vi "Page_Advanced_WriteAll.vi"(6 "ctl references":T1, 8 "error in (no error)":errorcluster, 11 "AB_InteropAssembly in":refnum<class "AB_InteropAssembly.lvclass">) -> (0 "error out":errorcluster, 3 "AB_InteropAssembly out":refnum<class "AB_InteropAssembly.lvclass">)   [LabVIEW 2020, in "AB_InteropAssembly.lvclass"]
uses:
  <vilib>/AppBuilder/AB_Classes/InteropAssembly/AB_InteropAssembly.lvclass
  <resource>/Framework/Providers/Builds/AppBuilder/AB_UI_Page_Advanced_References.ctl
  <vilib>/AppBuilder/AB_Classes/InteropAssembly/AB_InteropAssembly.lvclass/AB_InteropAssembly.ctl
  <vilib>/AppBuilder/AB_Classes/Application/AB_Application.lvclass
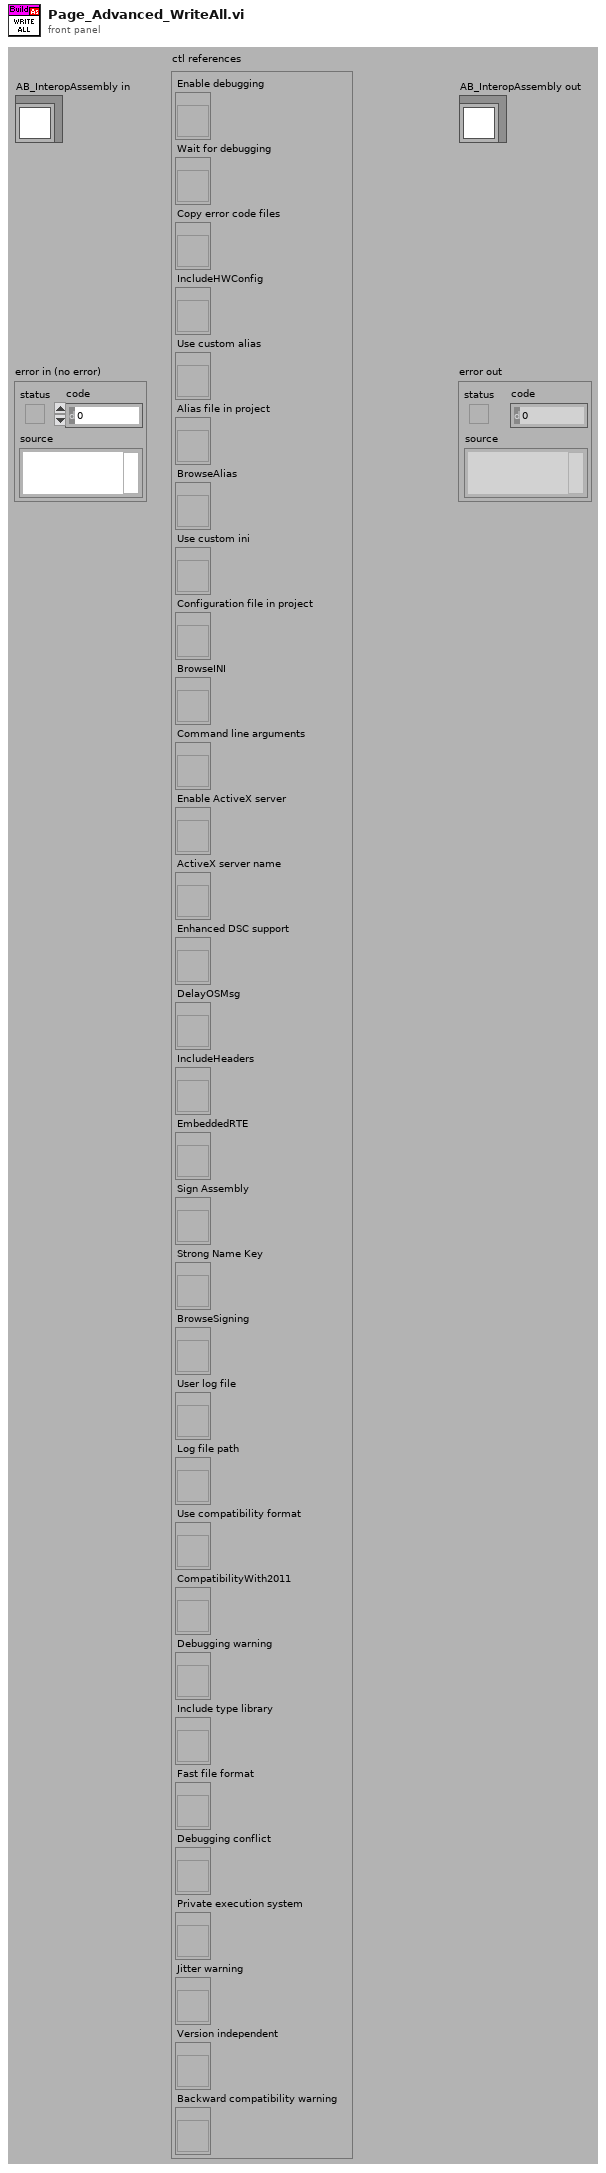
[diagram p1: front panel]
types:
  T1 = typedef "AB_UI_Page_Advanced_References.ctl" = cluster{"Enable debugging":refnum<vi>, "Wait for debugging":refnum<vi>, "Copy error code files":refnum<vi>, "IncludeHWConfig":refnum<vi>, "Use custom alias":refnum<vi>, "Alias file in project":refnum<vi>, "BrowseAlias":refnum<vi>, "Use custom ini":refnum<vi>, "Configuration file in project":refnum<vi>, "BrowseINI":refnum<vi>, "Command line arguments":refnum<vi>, "Enable ActiveX server":refnum<vi>, "ActiveX server name":refnum<vi>, "Enhanced DSC support":refnum<vi>, "DelayOSMsg":refnum<vi>, "IncludeHeaders":refnum<vi>, "EmbeddedRTE":refnum<vi>, "Sign Assembly":refnum<vi>, "Strong Name Key":refnum<vi>, "BrowseSigning":refnum<vi>, "User log file":refnum<vi>, "Log file path":refnum<vi>, "Use compatibility format":refnum<vi>, "CompatibilityWith2011":refnum<vi>, "Debugging warning":refnum<vi>, "Include type library":refnum<vi>, "Fast file format":refnum<vi>, "Debugging conflict":refnum<vi>, "Private execution system":refnum<vi>, "Jitter warning":refnum<vi>, "Version independent":refnum<vi>, "Backward compatibility warning":refnum<vi>}
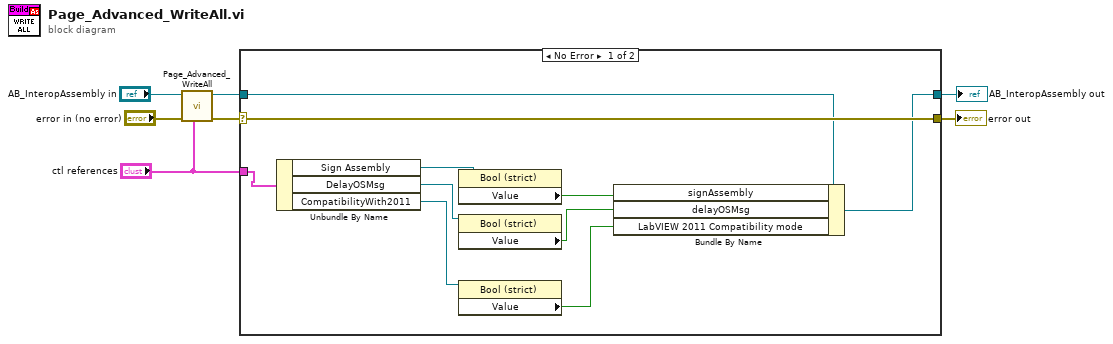
[diagram p0: block diagram]
diagram:
  n1 = call-parent "Page_Advanced_WriteAll.vi"("ctl references"="ctl references", "error in (no error)"="error in (no error)", "AB_Application in"="AB_InteropAssembly in") -> ("error out"=w6:errorcluster, "AB_Application out"=w5:refnum<class "AB_InteropAssembly.lvclass">)  [unwired: 7 out]
  n2 = case shown="No Error" w6 {
    selector: w6 -> [w17 w18]
    tunnel: w5 -> [w15 w19]
    tunnel: [w16 w19] -> w1
    tunnel: [w17 w18] -> w4
    tunnel: "ctl references" -> [w14 _]
    frame No Error {
      n3 = Unbundle By Name(w14) -> ("Sign Assembly"=w13:refnum<vi>, "DelayOSMsg"=w11:refnum<vi>, "CompatibilityWith2011"=w9:refnum<vi>)
      n4 = property class="Bool (strict)"(reference=w13) -> ("Value"=w12:bool)  [unwired: 1 in, 2 out]
      n5 = property class="Bool (strict)"(reference=w11) -> ("Value"=w10:bool)  [unwired: 1 in, 2 out]
      n6 = property class="Bool (strict)"(reference=w9) -> ("Value"=w8:bool)  [unwired: 1 in, 2 out]
      n7 = Bundle By Name(cluster=w15, "signAssembly"=w12, "delayOSMsg"=w10, "LabVIEW 2011 Compatibility mode"=w8) -> (w16:refnum<class "AB_InteropAssembly.lvclass">)
    }
    frame Error {
    }
  }
  "error out" <- w4
  "AB_InteropAssembly out" <- w1
